vi "Tenney Check Limits.vi"(5 "Temperature Average":dbl, 7 "Humidity Average":dbl, 8 "error in (no error)":errorcluster, 10 "Temperature Limits":T2={"Target Temperature Upper limit"=68.0, "Target Temperature Lower limit"=67.0, "Target Humidity Lower limit"=48.5, "Target Humidity Upper limit"=51.5, "Chamber Temperature Upper limit"=68.0, "Chamber Temperature Lower limit"=67.0, "Chamber Humidity Lower limit"=48.5, "Chamber Humidity Upper limit"=51.5, "Chamber Adjustment Increment (F)"=0.1, "Chamber Adjustment Interval (Minutes)"=10.0, "Chamber Adjustment Increment (%)"=0.1, "Chamber Adjustment Interval Fast (Minutes)"=5.0}, 11 "Tenney Environmental Chamber Data Output in":T1) -> (0 "error out":errorcluster, 1 "Data CMD":dbl[](array[numeric]), 2 "State CMD":string[](array[string]), 3 "Tenney Environmental Chamber Data Output":T1)   [LabVIEW 2023]
uses:
  controls/Tenney Temperature Limits.ctl
  Drivers/Tidal Engineering/Type Definitions/Tenney Environmental Chamber Data.ctl
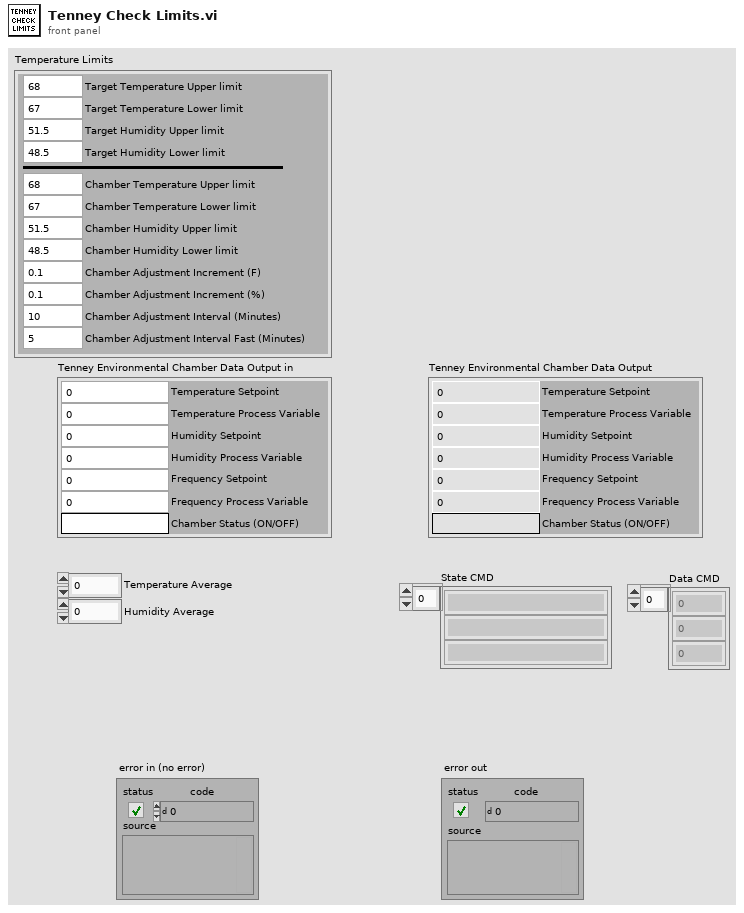
[diagram p1: front panel]
types:
  T1 = typedef "Tenney Environmental Chamber Data.ctl" = cluster{"Temperature Setpoint":dbl, "Temperature Process Variable":dbl, "Humidity Setpoint":dbl, "Humidity Process Variable":dbl, "Frequency Setpoint":dbl, "Frequency Process Variable":dbl, "Chamber Status (ON/OFF)":string}
  T2 = typedef "Tenney Temperature Limits.ctl" = cluster{"Target Temperature Upper limit":dbl, "Target Temperature Lower limit":dbl, "Target Humidity Lower limit":dbl, "Target Humidity Upper limit":dbl, "Chamber Temperature Upper limit":dbl, "Chamber Temperature Lower limit":dbl, "Chamber Humidity Lower limit":dbl, "Chamber Humidity Upper limit":dbl, "Chamber Adjustment Increment (F)":dbl, "Chamber Adjustment Interval (Minutes)":dbl, "Chamber Adjustment Increment (%)":dbl, "Chamber Adjustment Interval Fast (Minutes)":dbl}
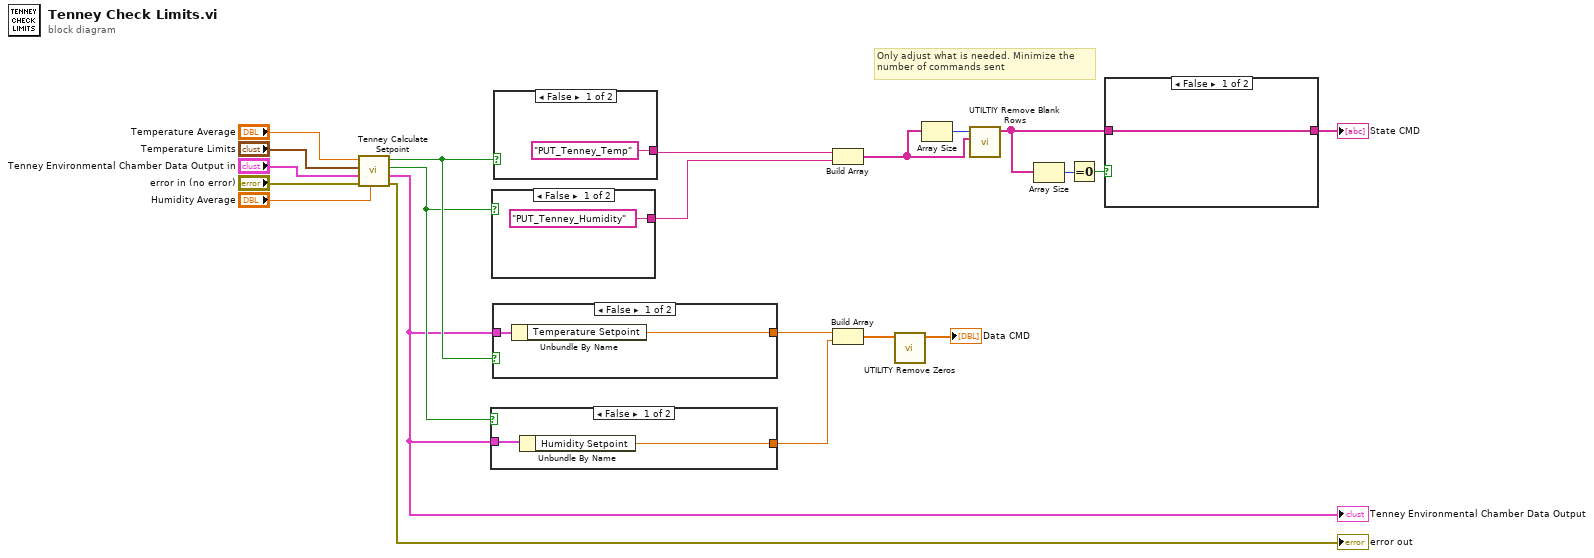
[diagram p0: block diagram]
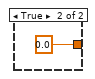
[diagram p2: hidden frame]
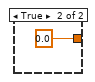
[diagram p3: hidden frame]
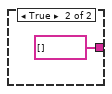
[diagram p4: hidden frame]
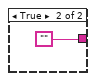
[diagram p5: hidden frame]
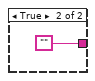
[diagram p6: hidden frame]
diagram:
  # "Only adjust what is needed. Minimize the\nnumber of commands sent"
  n1 = call "Tenney Calculate Setpoint.vi"("Humidity Average"="Humidity Average", "error in (no error)"="error in (no error)", "Tenney Environmental Chamber Data Input"="Tenney Environmental Chamber Data Output in", "Temperature Limits"="Temperature Limits", "Temperature Average"="Temperature Average") -> ("error out"=→"error out":errorcluster, "Tenney Environmental Chamber Data Output"=w5:T1, "Humidity In Range?"=w6:bool, "Temperature In Range?"=w7:bool)  [unwired: 3 in]
  "Tenney Environmental Chamber Data Output" <- w5
  n2 = case shown="False" w6 {
    tunnel: [w22 0.0] -> w3
    tunnel: w5 -> [w23 _]
    frame False {
      n3 = Unbundle By Name(w23) -> ("Humidity Setpoint"=w22:dbl)
    }
    frame True {
    }
  }
  n4 = case shown="False" w6 {
    tunnel: ["PUT_Tenney_Humidity" ("Message") ""] -> w21
    frame False {
    }
    frame True {
    }
  }
  n5 = case shown="False" w7 {
    tunnel: w5 -> [w28 _]
    tunnel: [w27 0.0] -> w4
    frame False {
      n6 = Unbundle By Name(w28) -> ("Temperature Setpoint"=w27:dbl)
    }
    frame True {
    }
  }
  n7 = case shown="False" w7 {
    tunnel: ["PUT_Tenney_Temp" ("Message") ""] -> w20
    frame False {
    }
    frame True {
    }
  }
  n8 = Build Array(w20, w21) -> (w16:string[])
  n9 = Build Array(w4, w3) -> (w2:dbl[])
  n10 = call "UTILITY Remove Zeros.vi"("Array in"=w2) -> ("Array out"=→"Data CMD":dbl[])  [unwired: 10 in]
  n11 = Array Size(array=w16) -> (size(s)=w17:i32)
  n12 = call "UTILTIY Remove Blank Rows.vi"("all rows in"=w16, "Numeric"=w17) -> ("all rows out"=w13:string[])  [unwired: 9 in]
  n13 = Array Size(array=w13) -> (size(s)=w15:i32)
  n14 = Equal To 0?(x=w15) -> (x = 0?=w14:bool)
  n15 = case shown="False" w14 {
    tunnel: w13 -> [w32 _]
    tunnel: [w32 string[] []] -> w12
    frame False {
    }
    frame True {
    }
  }
  "State CMD" <- w12
